vi "GetConstantReference.vi"(6 "error in":errorcluster, 9 "Constant in":refnum<class "Constant.lvclass">) -> (0 "error out":errorcluster, 1 "reference out":refnum<vi>, 3 "Constant out":refnum<class "Constant.lvclass">)   [LabVIEW 2014, in "Raspberry Pi Compatible Compiler for LabVIEW.lvlib" / "Constant.lvclass"]
uses:
  Constant.lvclass
  Generic/Generic.lvclass
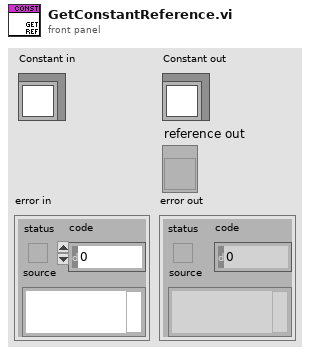
[diagram p1: front panel]
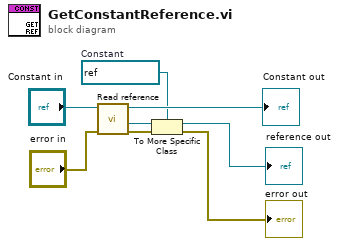
[diagram p0: block diagram]
diagram:
  w4 = refnum<vi> refnum  # Constant
  n1 = call "Read reference.vi"("error in"="error in", "GObject in"="Constant in") -> ("error out"=w5:errorcluster, "reference"=w6:refnum<vi>, "GObject out"=→"Constant out":refnum<class "Constant.lvclass">)  [unwired: 5 in]
  n2 = To More Specific Class(target class=w4, reference=w6, error in=w5) -> (specific class reference=→"reference out":refnum<vi>, error out=→"error out":errorcluster)
